vi "Analyze.vi"(6 "error in":errorcluster, 8 "n-channel data (2D DBL)":dbl[][](array[numeric])) -> (0 "error out":errorcluster, 2 "message":string)   [LabVIEW 2020]
uses:
  <vilib>/Analysis/5stat.llb/RMS (DBL).vi
  <vilib>/Analysis/NI_AALPro.lvlib
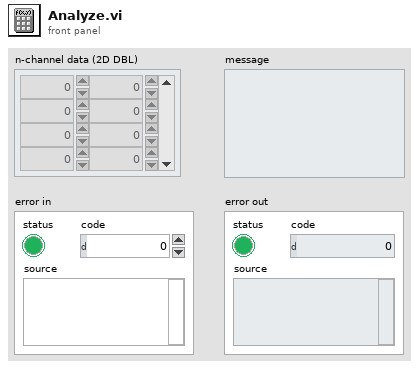
[diagram p1: front panel]
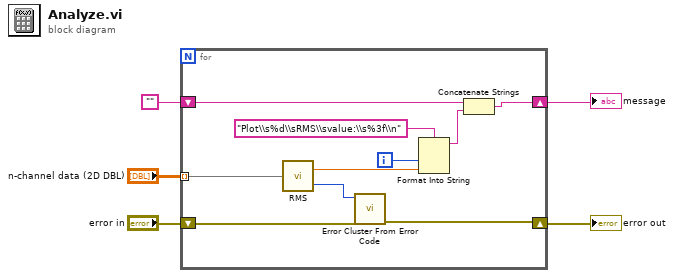
[diagram p0: block diagram]
diagram:
  n1 = for {
    tunnel: "n-channel data (2D DBL)" -> [w15] mode=indexing
    shift-right: [w9] -> w5
    shift-left: "" -> [w10]
    shift-right: [w6] -> w1
    shift-left: "error in" -> [w7]
    i -> [w14]
    n2 = call-poly <vilib>:"RMS.vi"("X"=w15) -> ("rms value"=w13:dbl, "error"=w8:i32)
    n3 = call <vilib>:"Error Cluster From Error Code.vi"("error in (no error)"=w7, "error code (0)"=w8) -> ("error out"=w6:errorcluster)  [unwired: 7 in]
    n4 = Format Into String(format string="Plot\\s%d\\sRMS\\svalue:\\s%3f\\n", w14, w13) -> (resulting string=w11:string)  [unwired: 2 in, 1 out]
    n5 = Concatenate Strings(w10, w11) -> (w9:string)
  }
  "message" <- w5
  "error out" <- w1
